vi "Reset Force.vi"(8 "error in (no error)":errorcluster, 11 "Model in":refnum<class "Model.lvclass">) -> (0 "error out":errorcluster, 3 "Model out":refnum<class "Model.lvclass">)   [LabVIEW 2016]
uses:
  Modbus/DesktopModbus/DesktopModbus.lvclass
  Common_RT_FAILC/FAILC/FAILC.lvclass
  Model.lvclass
  C:/CODE/ts_HPMT/Common_RT_ILC/ILC/ILC.lvclass
  C:/CODE/ts_HPMT/Common_RT_Modbus/IModbus/IModbus.lvclass
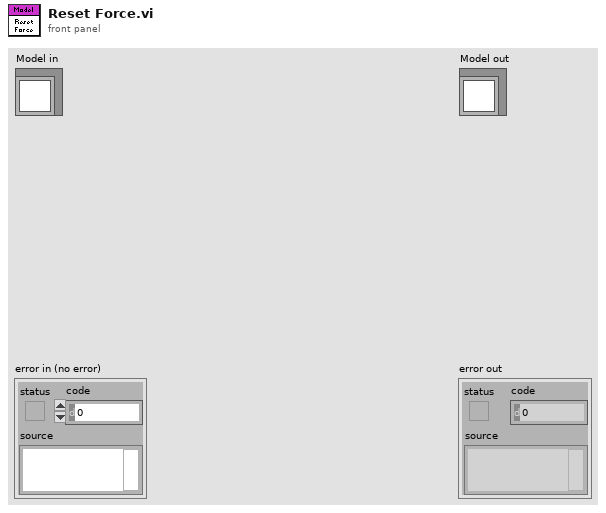
[diagram p1: front panel]
types:
  T1 = typedef "RTHPILC.lvlib/HPData.ctl" = cluster{"Constants":T2, "Command":T3, "Telemetry":T4, "Responses":T5, "Timings":T7}
  T2 = typedef "RTHPILC.lvlib/HPConstants.ctl" = cluster{"ID":i16}
  T3 = typedef "RTHPILC.lvlib/HPCommand.ctl" = cluster{"AxialSetPoint":i32, "LateralSetPoint":i32, "AxialBoosterValveGain":sgl, "LateralBoosterValveGain":sgl}
  T4 = typedef "RTHPILC.lvlib/HPTelemetry.ctl" = cluster{"ILCFault":bool, "BroadcastCounter":u8, "AxialLoadCellForce":sgl, "LateralLoadCellForce":sgl, "AxialBoosterValveGain":sgl, "LateralBoosterValveGain":sgl}
  T5 = typedef "RTHPILC.lvlib/HPResponses.ctl" = cluster{"BoosterValveGain":T6, "ReadBoosterValveGain":T6, "SetForce":T6, "ForceAndStatus":T6}
  T6 = typedef "RTModbus.lvlib/ExceptionCodes.ctl" = u16
  T7 = typedef "RTHPILC.lvlib/HPTimings.ctl" = cluster{"BroadcastSetForce":u32, "BoosterValveGain":u32, "FreezeSensorValues":u32, "ForceAndStatus":u32, "ReadBoosterValveGain":u32, "SetForce":u32}
  T8 = typedef "RTModbus.lvlib/TxFrame.ctl" = cluster{"Data":u8[], "WaitForTrigger":bool, "WaitForRx":u16, "TriggerIRQ":bool, "DelayMicroseconds":u16, "DelayMilliseconds":u16, "Timestamp":bool}
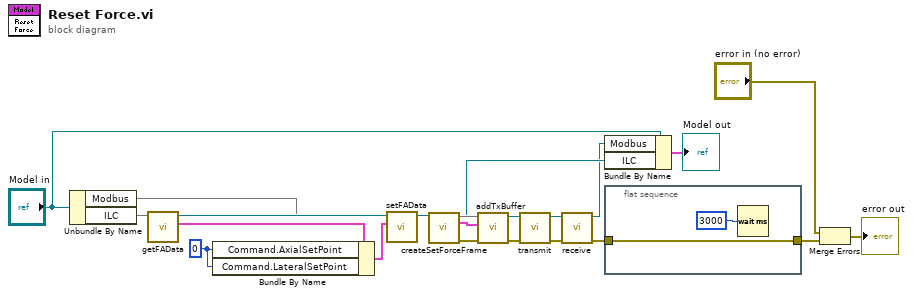
[diagram p0: block diagram]
diagram:
  w17 = 0 ("FACommand.AxialSetPoint")
  n1 = Unbundle By Name("Model in") -> ("Modbus"=w8, "ILC"=w7)
  n2 = call "getFAData.vi"("FAILC in"=w7) -> ("FAData"=w19:T1, "FAILC out"=w16:refnum<class "FAILC.lvclass">)  [unwired: 9 in]
  n3 = Bundle By Name(cluster=w19, "Command.AxialSetPoint"=w17, "Command.LateralSetPoint"=w17) -> (w18:T1)
  n4 = call "setFAData.vi"("FAData"=w18, "FAILC in"=w16) -> ("FAILC out"=w15:refnum<class "FAILC.lvclass">)  [unwired: 9 in]
  n5 = call-dynamic "createSetForceFrame.vi"("FAILC in"=w15) -> ("FAILC out"=w4:refnum<class "FAILC.lvclass">, "TxFrame"=w14:T8, "error out"=w13:errorcluster)  [unwired: 12 in]
  n6 = call-dynamic "addTxBuffer.vi"("error in (no error)"=w13, "TxFrame"=w14, "DesktopModbus in"=w8) -> ("error out"=w12:errorcluster, "DesktopModbus out"=w9:refnum<class "DesktopModbus.lvclass">)  [unwired: 7 in]
  n7 = call-dynamic "transmit.vi"("error in (no error)"=w12, "DesktopModbus in"=w9) -> ("error out"=w11:errorcluster, "DesktopModbus out"=w10:refnum<class "DesktopModbus.lvclass">)  [unwired: 8 in]
  n8 = call-dynamic "receive.vi"("error in (no error)"=w11, "DesktopModbus in"=w10) -> ("error out"=w1:errorcluster, "DesktopModbus out"=w3:refnum<class "DesktopModbus.lvclass">)  [unwired: 7 in, 1 out]
  n9 = Bundle By Name(cluster="Model in", "Modbus"=w3, "ILC"=w4) -> (→"Model out":cluster{})
  n10 = flat-sequence {
    tunnel: [w22] -> w2
    tunnel: w1 -> [w22]
    frame #0 {
      n11 = Wait (ms)(milliseconds to wait=u32 3000) -> ()  [unwired: 1 out]
    }
  }
  n12 = Merge Errors("error in (no error)", w2) -> (→"error out":errorcluster)
